vi "Ivium driver 1-03 - Copy2.vi"() -> ()   [LabVIEW 2020]
uses:
  Users/Benjamin/Desktop/StateMachine/Documents/LabVIEW Data/transmittance/controls/State.ctl
  IVIUM_remdriver.lvlib
panel:
  in  "Get device status 2":bool
  in  "Tab Control Ac/external/bistat":enum32{"AC", "Extern", "BiStat"}(tab)
  in  "Record I":bool
  in  "Read and set values":bool
  in  "Exit and disconnect":bool
  out "Values to re-intialise to at end\nof the measument":T1
  out "Device serial number":string
  in  "Read device serial number":bool
  in  "Tab Control direct mode/method mode":enum32{"Direct Control", "Method control"}(tab)
  out "cell on":bool
  in  "Set Mux channel":i32
  in  "Get current":bool
  out "current":dbl caption="A" format="%_4g"
  in  "cell potential":dbl caption="V" format="%_3p"
  in  "Apply":enum16{"off", "on"}(ring)
  in  "Current range":T2(ring)=enum."10 mA"
  in  "Configuration":T3(ring)
  out "Device Status indicator":string
  in  "Get device status":bool
  out "cell-off button pressed":bool
  out "E_overload":bool
  out "Aninput1_overload":bool
  out "I_overload":bool
  in  "Get cell status":bool
  in  "Reset 2":bool
  out "potential":dbl caption="V" format="%_4g"
  in  "Get potential":bool
  in  "Set Filter":T4(ring)=enum."10 kHz"
  in  "Set Stability":T5(ring)=enum."Standard"
  in  "Reset 3":bool
  in  "stop":bool
  # "Ac signal"
  # "Analog input"
  # "Digital output"
  # "Analog output"
  # "ch1"
  # "ch2"
  # "ch3"
  # "ch4"
  # "ch5"
  # "Digital input"
  # "ch6"
  # "ch7"
  # "ch8"
  # "I overload"
  # "Cell-off button pressed"
  # "E overload"
  # "Aninput1 overload"
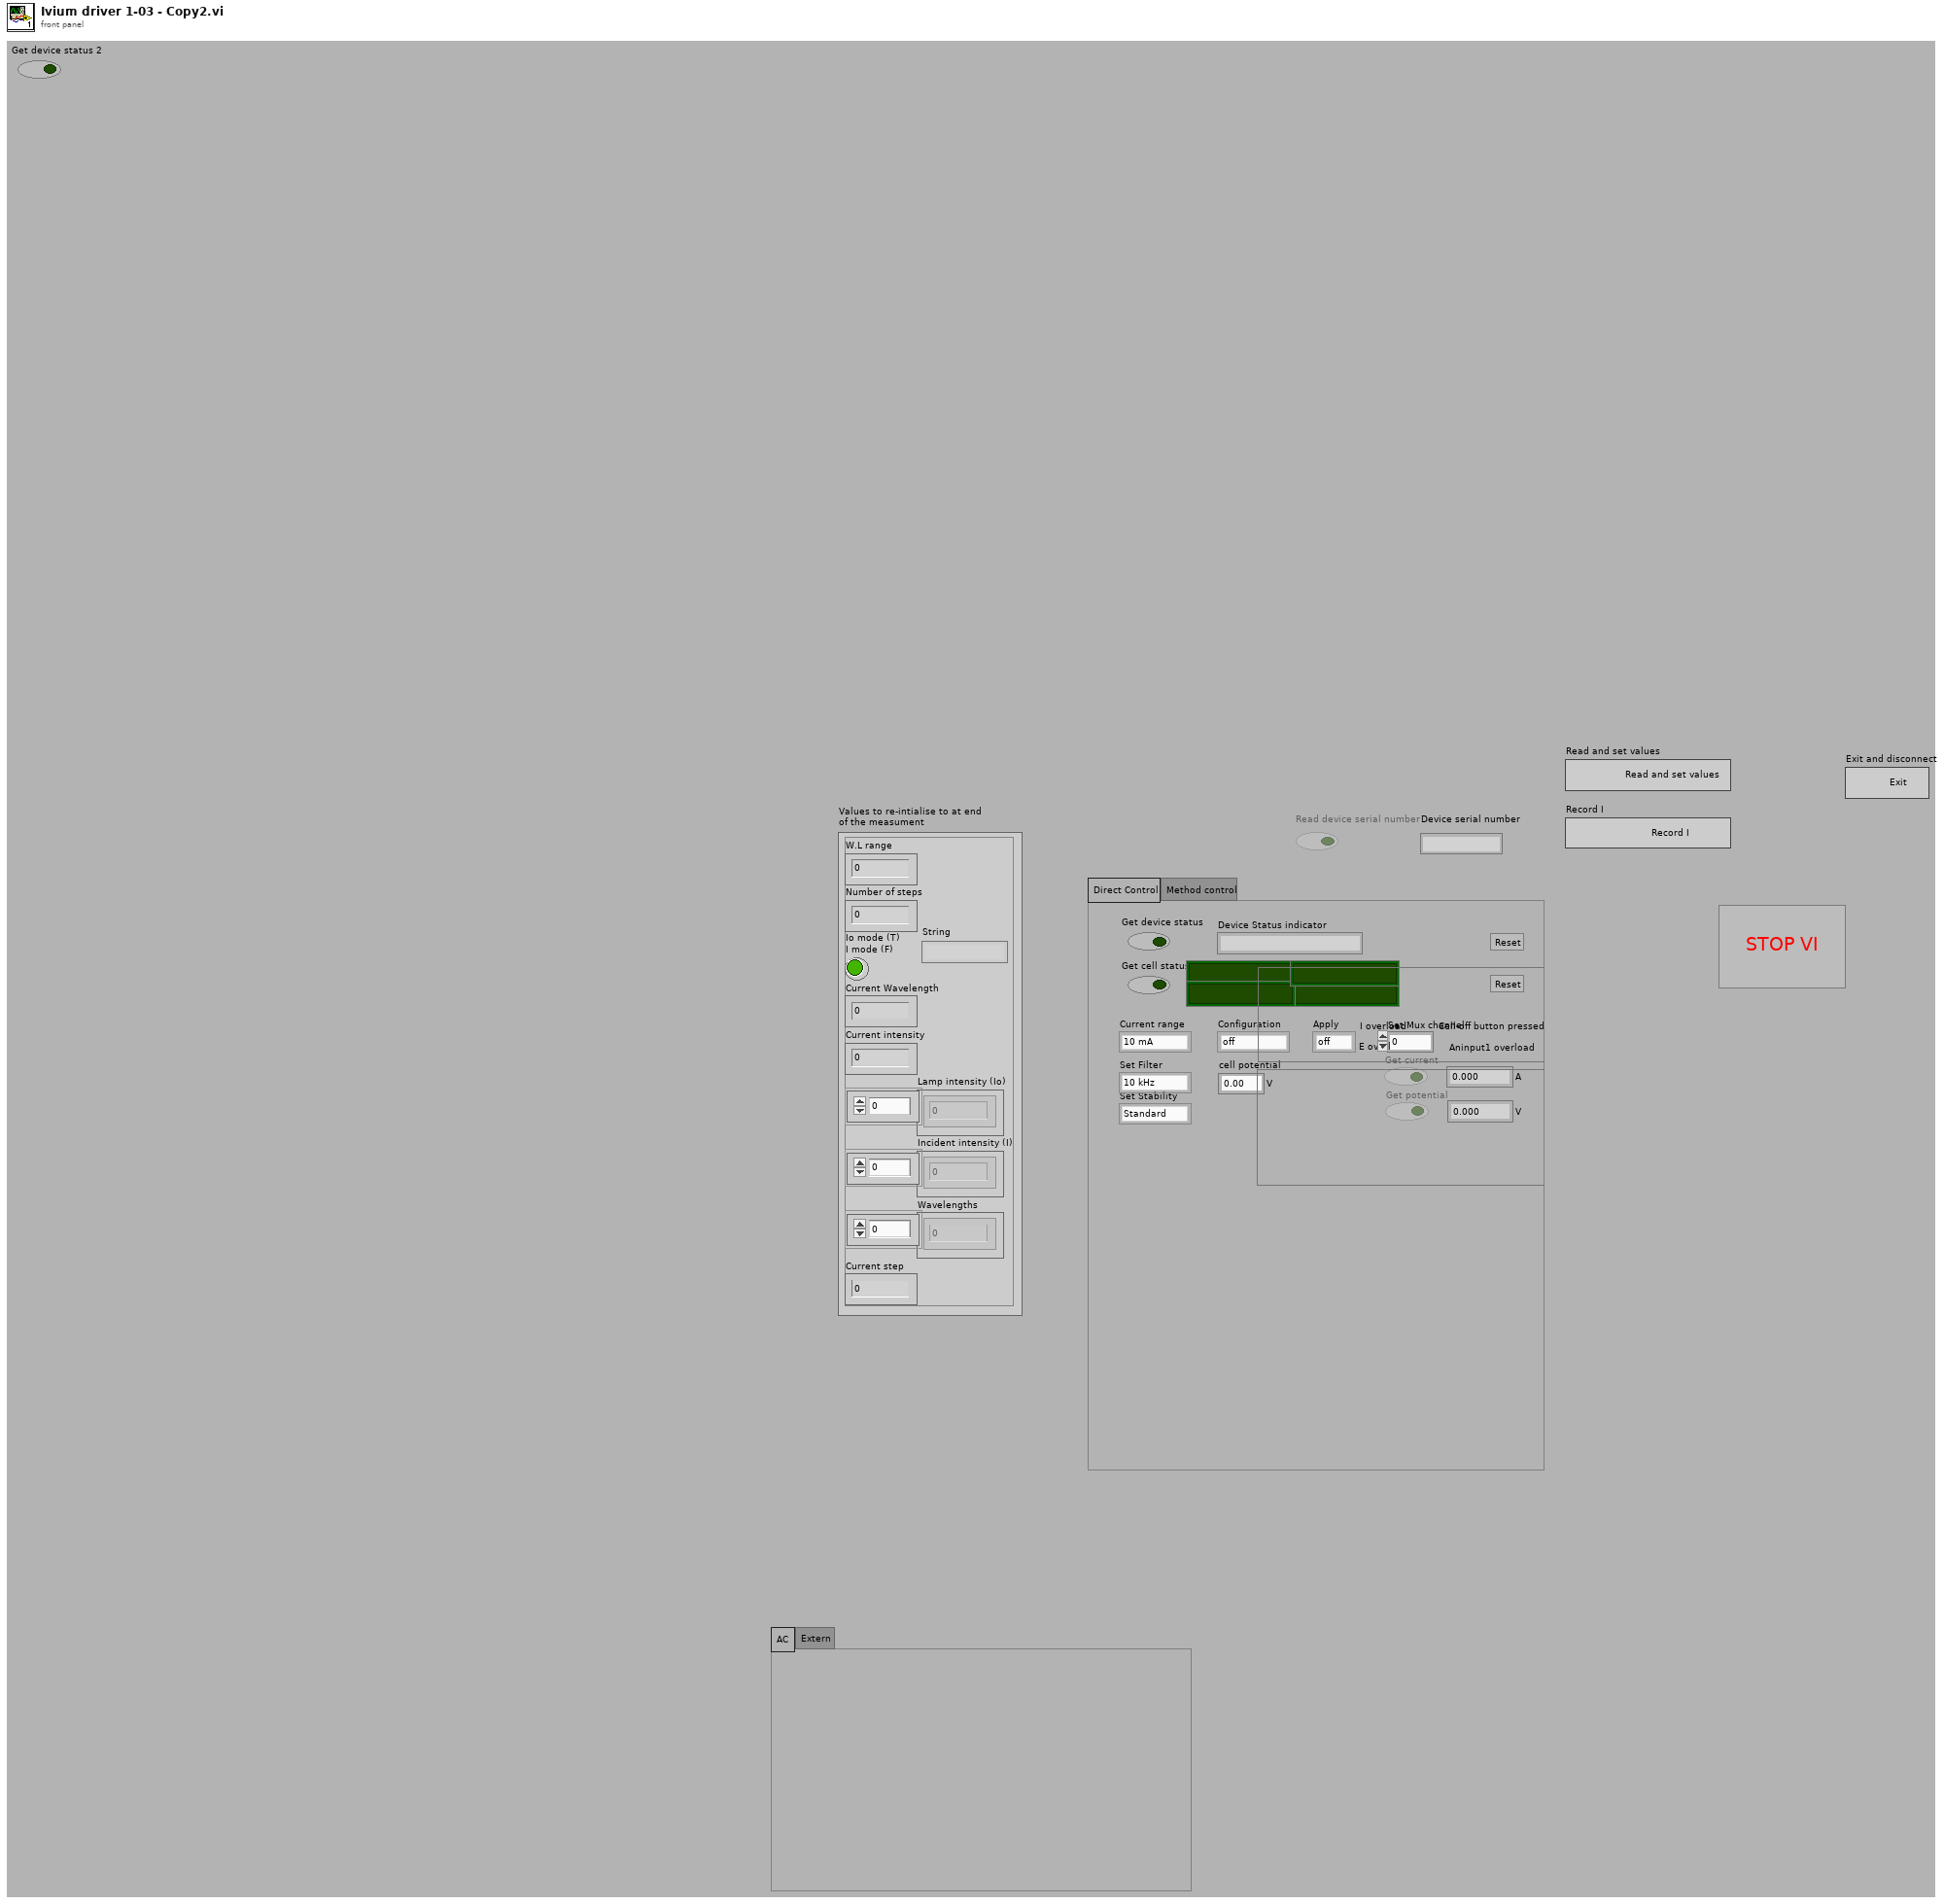
[diagram p1: front panel]
types:
  T1 = cluster{"W.L range":dbl, "Number of steps":dbl, "Io mode (T) \nI mode (F)":bool, "Current Wavelength":dbl, "Current intensity":dbl, "Lamp intensity (Io)":dbl[], "Incident intensity (I) ":dbl[], "Wavelengths ":dbl[], "Current step":dbl, "String":string}
  T2 = enum16{"10 A", "1 A", "100 mA", "10 mA", "1 mA", "100 uA", "10 uA", "1 uA", "100 nA", "10 nA", "1 nA", "100 pA", "10 pA", "1 pA"}
  T3 = enum16{"off", "EStat4EL", "EStat2EL", "EStatDummy1", "EStatDummy2", "EStatDummy3", "EStatDummy4", "IStat4EL", "IStat2EL", "IStatDummy", "BiStat4EL", "BiStat2EL"}
  T4 = enum16{"1 MHz", "100 kHz", "10 kHz", "1 kHz", "10 Hz"}
  T5 = enum16{"High Speed", "Standard", "High Stability"}
  T6 = cluster{"W.L range":dbl, "Number of steps":dbl, "Io mode (T) \nI mode (F)":bool, "Current Wavelength":dbl, "Current intensity":dbl, "Lamp intensity (Io)":dbl[], "Incident intensity (I) ":dbl[], "Wavelengths ":dbl[], "Current step":dbl, "Status":string}
  T7 = typedef "State.ctl" = enum16{"Initialize", "Wait for Event", "Update and read", "Close ", "Output data and process", "Exit"}
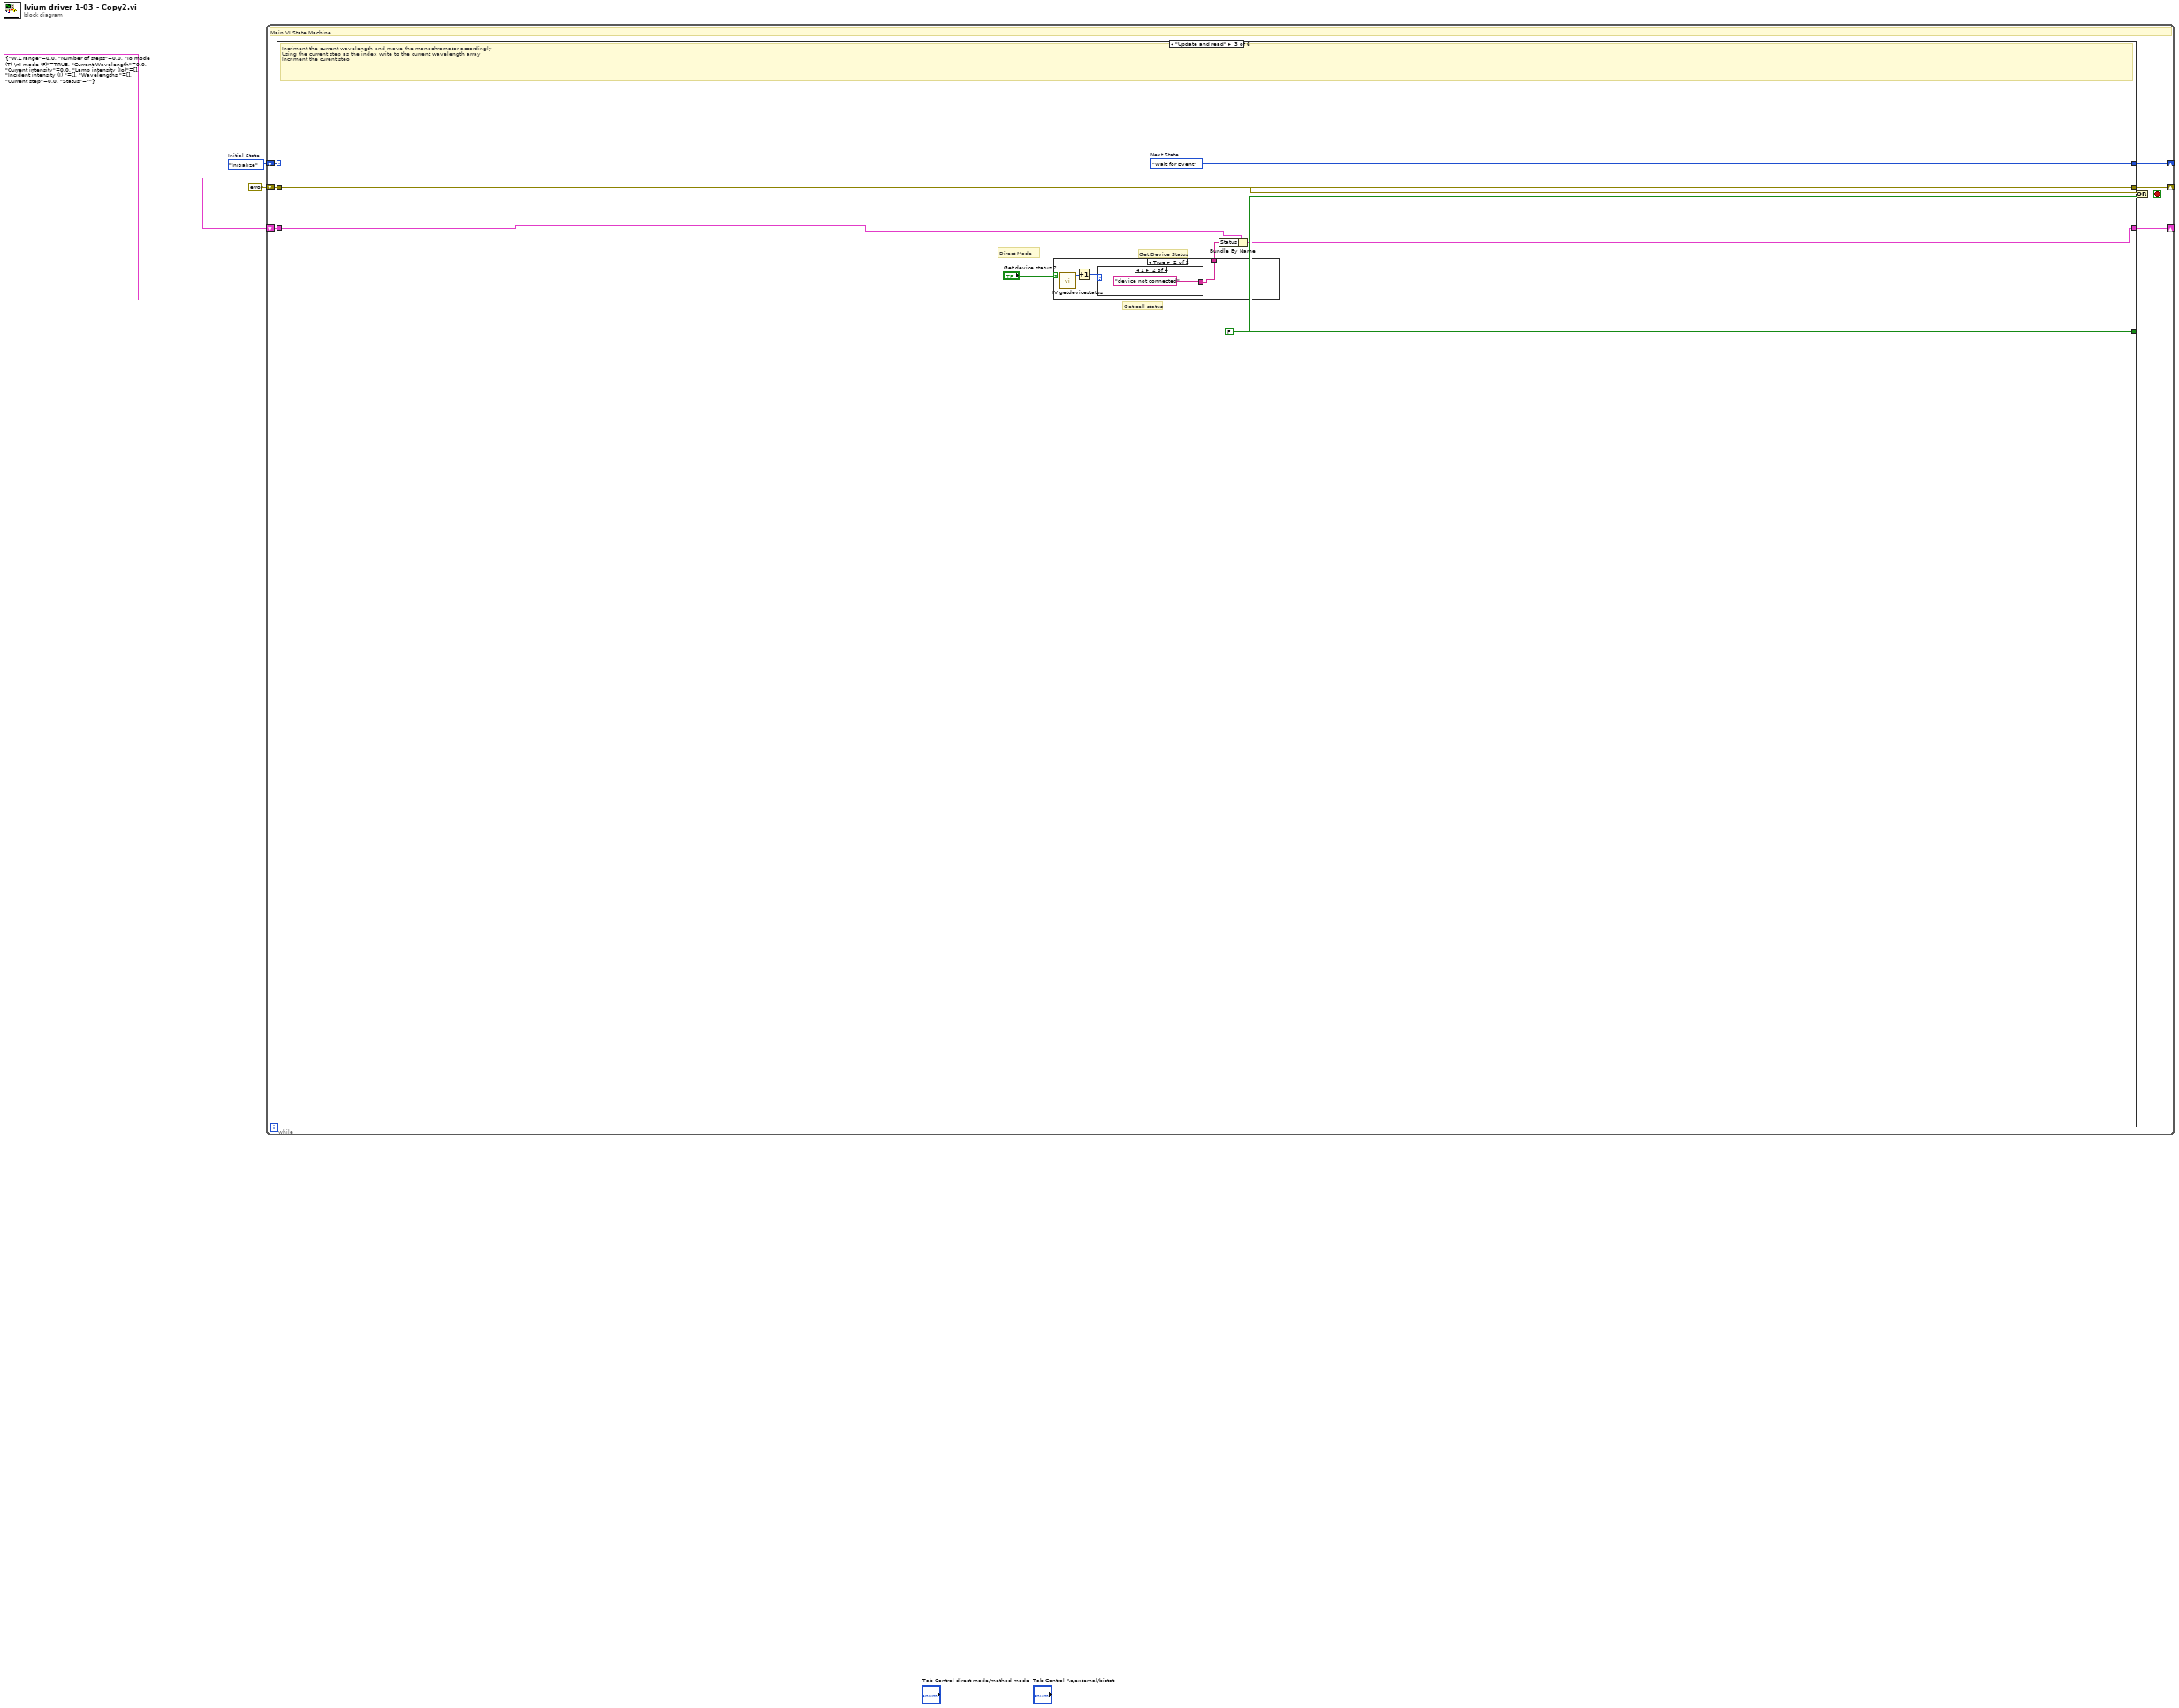
[diagram p0: block diagram]
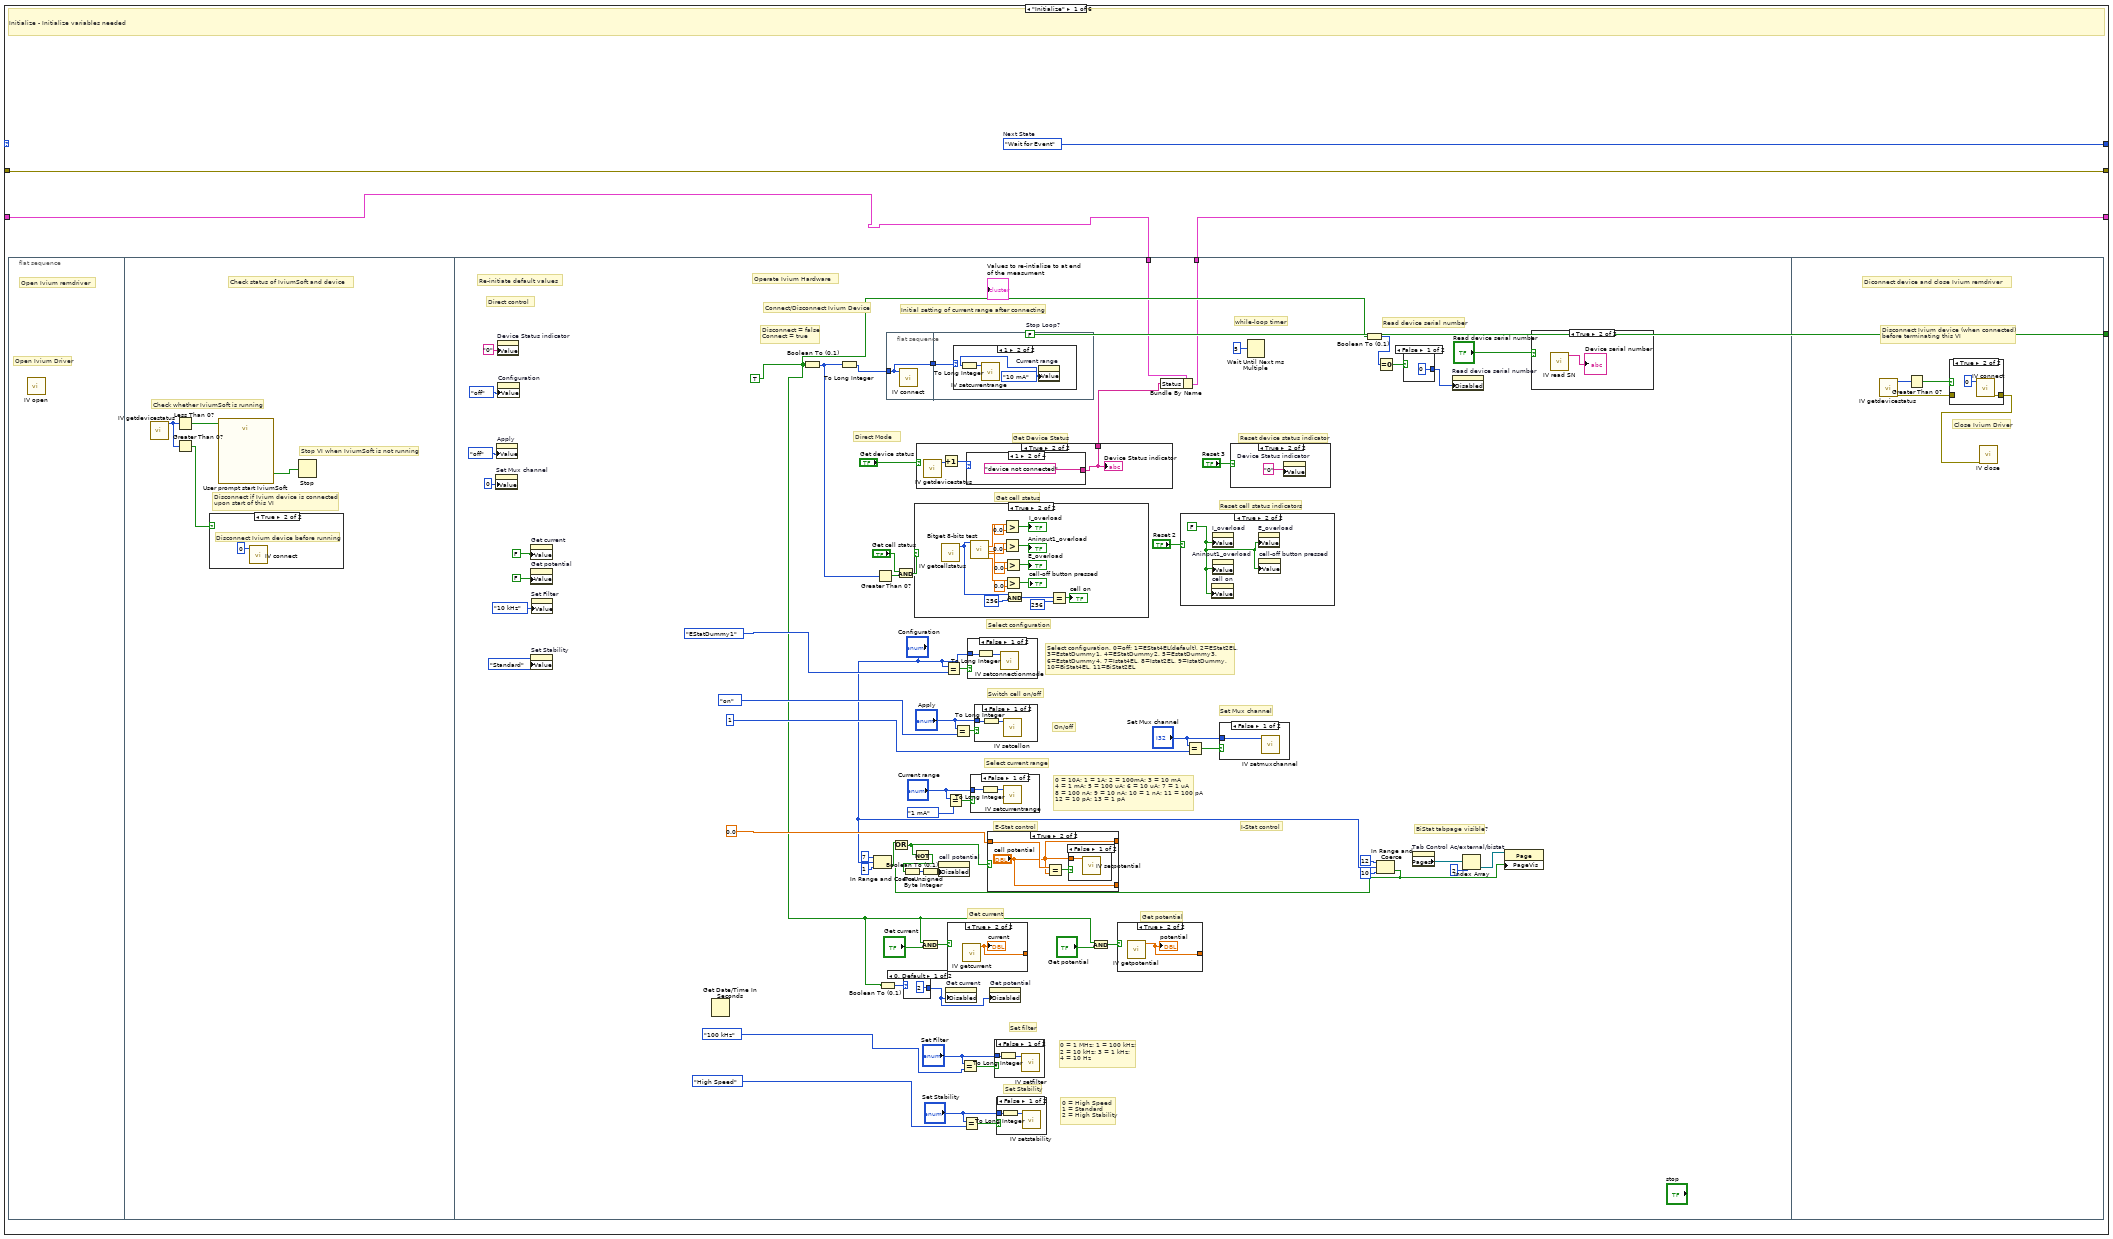
[diagram p2: hidden frame]
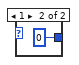
[diagram p5: hidden frame]
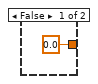
[diagram p10: hidden frame]
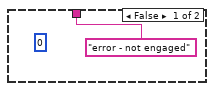
[diagram p13: hidden frame]
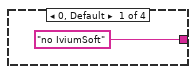
[diagram p14: hidden frame]
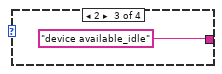
[diagram p15: hidden frame]
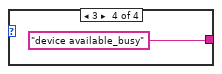
[diagram p16: hidden frame]
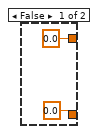
[diagram p17: hidden frame]
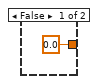
[diagram p19: hidden frame]
diagram:
  w3 = State."Initialize"  # Initial State
  n1 = while {
    shift-right: [w10] -> _
    shift-left: w3 -> [w11]
    shift-right: [w8] -> _
    shift-left: T6 {"W.L range"=0.0, "Number of steps"=0.0, "Io mode (T) \nI mode (F)"=TRUE, "Current Wavelength"=0.0, "Current intensity"=0.0, "Lamp intensity (Io)"=[], "Incident intensity (I) "=[], "Wavelengths "=[], "Current step"=0.0, "Status"=""} -> [w9]
    shift-right: [w4] -> _
    shift-left: errorcluster {"status"=FALSE, "code"=0, "source"=""} ("error constant") -> [w7]
    stop <- w5 stop-if-true
    # "Main VI State Machine"
    n2 = case shown="\"Update and read\"" w11 {
      tunnel: [w16 w155 w175 w192 State."Exit" ("f") State."Wait for Event" ("f")] -> w10
      tunnel: [w15 w154 FALSE ("Stop Loop?") w190 _ _] -> w6
      tunnel: w9 -> [w12 w151 w171 w191 w198 _]
      tunnel: [w13 w150 w169 w191 w198 w199] -> w8
      tunnel: w7 -> [w14 w153 w173 w185 w197 w201]
      tunnel: [w14 w152 w173 w184 w197 w201] -> w4
      frame "Initialize" {
        w15 = FALSE  # Stop Loop?
        w16 = State."Wait for Event"  # Next State
        # "Initialize - Initialize variables needed"
        n3 = flat-sequence {
          tunnel: w12 -> [w24]
          tunnel: [w22] -> w13
          frame #0 {
            # "Open Ivium Driver"
            # "Open Ivium remdriver"
            n4 = call "IV open.vi"() -> ()  [unwired: 10 in, 2 out]
          }
          frame #1 {
            # "Check status of IviumSoft and device"
            # "Stop VI when IviumSoft is not running"
            # "Disconnect if Ivium device is connected \nupon start of this VI"
            # "Check whether IviumSoft is running"
            n5 = call "IV getdevicestatus.vi"() -> ("return type"=w20:i32)  [unwired: 10 in, 1 out]
            n6 = Less Than 0?(x=w20) -> (x < 0?=w17:bool)
            n7 = Greater Than 0?(x=w20) -> (x > 0?=w19:bool)
            n8 = case shown="True" w19 {
              frame False {
              }
              frame True {
                # "Disconnect Ivium device before running"
                n9 = call "IV connect.vi"("devconnect"=0) -> ()  [unwired: 8 in, 3 out]
              }
            }
            n10 = call "User prompt start IviumSoft.vi"("Enable"=w17) -> ("OK"=w18:bool)  [unwired: 17 in, 1 out]
            n11 = Stop(stop? (T)=w18) -> ()
          }
          frame #2 {
            w26 = TRUE ("Boolean")
            # "BiStat tabpage visible?"
            # "Get potential"
            # "Get current"
            # "Set Mux channel"
            # "Reset device status indicator"
            # "0 = High Speed\n1 = Standard \n2 = High Stability"
            # "Set Stability"
            # "0 = 1 MHz; 1 = 100 kHz; \n2 = 10 kHz; 3 = 1 kHz; \n4 = 10 Hz"
            # "Set filter"
            # "On/off"
            # "I-Stat control"
            # "E-Stat control"
            # "Reset cell status indicators"
            # "Get cell status"
            # "Get Device Status"
            # "0 = 10A; 1 = 1A; 2 = 100mA; 3 = 10 mA\n4 = 1 mA; 5 = 100 uA; 6 = 10 uA; 7 = 1 uA\n8 = 100 nA; 9 = 10 nA; 10 = 1 nA; 11 = 100 pA\n12 = 10 pA; 13 = 1 pA"
            # "Select configuration"
            # "Direct Mode"
            # "Switch cell on/off"
            # "Select current range"
            # "Select configuration, 0=off; 1=EStat4EL(default), 2=EStat2EL, 3=EstatDummy1, 4=EStatDummy2, 5=EstatDummy3, 6=EstatDummy4, 7=Istat4EL, 8=Istat2EL, 9=IstatDummy, 10=BiStat4EL, 11=BiStat2EL"
            # "Read device serial number"
            # "while-loop timer"
            # "Initial setting of current range after connecting"
            # "Disconnect = false\nConnect = true"
            # "Connect/Disconnect Ivium Device"
            # "Direct control"
            # "Re-initiate default values"
            # "Operate Ivium Hardware"
            n12 = property on="Set Mux channel" class="DigNum (strict)"("Value"=0 ("Set Mux channel")) -> ()  [unwired: 2 in, 2 out]
            n13 = property on="Apply" class="Enum (strict)"("Value"=enum16{"off", "on"}."off" ("Cell on/off")) -> ()  [unwired: 2 in, 2 out]
            n14 = property on="Device Status indicator" class="Str"("Value"="0" ("Device Status indicator 2")) -> ()  [unwired: 2 in, 2 out]
            n15 = property on="Configuration" class="Enum (strict)"("Value"=T3."off" ("Configuration")) -> ()  [unwired: 2 in, 2 out]
            n16 = property on="Get current" class="Bool (strict)"("Value"=FALSE ("Get current")) -> ()  [unwired: 2 in, 2 out]
            n17 = property on="Get potential" class="Bool (strict)"("Value"=FALSE ("Get potential")) -> ()  [unwired: 2 in, 2 out]
            n18 = property on="Set Stability" class="Enum (strict)"("Value"=T5."Standard" ("Set Stability")) -> ()  [unwired: 2 in, 2 out]
            n19 = property on="Set Filter" class="Enum (strict)"("Value"=T4."10 kHz" ("Set Filter")) -> ()  [unwired: 2 in, 2 out]
            n20 = Get Date/Time In Seconds() -> ()  [unwired: 1 out]
            n21 = Boolean To (0,1)(Boolean=w26) -> (0, 1=w69:i16)
            n22 = To Long Integer(number=w69) -> (32bit integer=w70:i32)
            n23 = In Range and Coerce(upper limit=u16 7, x="Configuration", lower limit=u16 1) -> (In Range?=w47:bool)  [unwired: 1 out]
            n24 = Greater Than 0?(x=w69) -> (x > 0?=w51:bool)
            n25 = Boolean To (0,1)(Boolean=w26) -> (0, 1=w39:i16)
            n26 = flat-sequence {
              tunnel: w70 -> [w86]
              tunnel: [w86] -> w25
              tunnel: w25 -> [w87]
              frame #0 {
                n27 = call "IV connect.vi"("devconnect"=w86) -> ()  [unwired: 8 in, 3 out]
              }
              frame #1 {
                n28 = case shown="1" w87 {
                  frame 0, Default {
                  }
                  frame 1 {
                    w88 = T2."10 mA" ("Current range selector")
                    n29 = To Long Integer(number=w88) -> (32bit integer=w89:i32)
                    n30 = call "IV setcurrentrange.vi"("value"=w89) -> ()  [unwired: 8 in, 3 out]
                    n31 = property on="Current range" class="Enum (strict)"("Value"=w88) -> ()  [unwired: 2 in, 2 out]
                  }
                }
              }
            }
            n32 = And(x="Get cell status", y=w51) -> (x .and. y?=w53:bool)
            n33 = case shown="0, Default" w39 {
              tunnel: [u8 2 u8 0] -> w38
              frame 0, Default {
              }
              frame 1 {
              }
            }
            n34 = case shown="True" w53 {
              frame False {
              }
              frame True {
                n35 = call "IV getcellstatus.vi"() -> ("devcellstatus out"=w105:i32)  [unwired: 9 in, 2 out]
                n36 = call "Bitget 8-bits test.vi"("x"=w105) -> ("c"=w110:dbl, "e"=w108:dbl, "f"=w109:dbl, "h"=w106:dbl)  [unwired: 19 in, 4 out]
                n37 = Greater?(x=w110, y=0.0) -> (0:→"I_overload":bool)
                n38 = Greater?(x=w108, y=0.0) -> (0:→"Aninput1_overload":bool)
                n39 = Greater?(x=w109, y=0.0) -> (0:→"E_overload":bool)
                n40 = Greater?(x=w106, y=0.0) -> (0:→"cell-off button pressed":bool)
                n41 = And(x=w105, y=256) -> (x .and. y?=w103:i32)
                n42 = Equal?(x=w103, y=256) -> (x = y?=→"cell on":bool)
              }
            }
            n43 = case shown="True" "Get device status" {
              tunnel: ["error - not engaged" w119] -> w23
              frame False {
                (unwired) 0
              }
              frame True {
                n44 = call "IV getdevicestatus.vi"() -> ("return type"=w121:i32)  [unwired: 10 in, 1 out]
                n45 = Increment(x=w121) -> (x+1=w120:i32)
                n46 = case shown="1" w120 {
                  tunnel: ["no IviumSoft" "device not connected" "device available_idle" "device available_busy"] -> w119
                  frame 0, Default {
                  }
                  frame 1 {
                  }
                  frame 2 {
                  }
                  frame 3 {
                  }
                }
                "Device Status indicator" <- w119
              }
            }
            n47 = And(x=w26, y="Get current") -> (x .and. y?=w60:bool)
            n48 = Equal?(x="Configuration", y=T3."EStatDummy1" ("Configuration")) -> (x = y?=w63:bool)
            n49 = property on="Get current" class="Bool (strict)"("Disabled"=w38) -> ()  [unwired: 2 in, 2 out]
            n50 = Equal?(x="Current range", y=T2."1 mA") -> (x = y?=w64:bool)
            n51 = case shown="True" w60 {
              tunnel: [0.0 ("value out") w133] -> _
              frame False {
              }
              frame True {
                n52 = call "IV getcurrent.vi"() -> ("value out"=w133:dbl)  [unwired: 9 in, 2 out]
                "current" <- w133
              }
            }
            n53 = Equal?(x="Apply", y=enum16{"off", "on"}."on" ("Apply")) -> (x = y?=w62:bool)
            n54 = Equal?(x="Set Filter", y=T4."100 kHz" ("Set Filter")) -> (x = y?=w31:bool)
            n55 = Equal?(x="Set Stability", y=T5."High Speed" ("Set Stability")) -> (x = y?=w44:bool)
            n56 = case shown="False" w63 {
              tunnel: "Configuration" -> [w136 _]
              frame False {
                n57 = To Long Integer(number=w136) -> (32bit integer=w137:i32)
                n58 = call "IV setconnectionmode.vi"("value"=w137) -> ()  [unwired: 8 in, 3 out]
              }
              frame True {
              }
            }
            n59 = case shown="False" w64 {
              tunnel: "Current range" -> [w138 _]
              frame False {
                n60 = To Long Integer(number=w138) -> (32bit integer=w139:i32)
                n61 = call "IV setcurrentrange.vi"("value"=w139) -> ()  [unwired: 8 in, 3 out]
              }
              frame True {
              }
            }
            n62 = case shown="False" w62 {
              tunnel: "Apply" -> [w134 _]
              frame False {
                n63 = To Long Integer(number=w134) -> (32bit integer=w135:i32)
                n64 = call "IV setcellon.vi"("cellon"=w135) -> ()  [unwired: 8 in, 3 out]
              }
              frame True {
              }
            }
            n65 = property on="Get potential" class="Bool (strict)"("Disabled"=w38) -> ()  [unwired: 2 in, 2 out]
            n66 = case shown="False" w31 {
              tunnel: "Set Filter" -> [w97 _]
              frame False {
                n67 = To Long Integer(number=w97) -> (32bit integer=w96:i32)
                n68 = call "IV setfilter.vi"("value"=w96) -> ()  [unwired: 8 in, 3 out]
              }
              frame True {
              }
            }
            n69 = case shown="False" w44 {
              tunnel: "Set Stability" -> [w95 _]
              frame False {
                n70 = To Long Integer(number=w95) -> (32bit integer=w94:i32)
                n71 = call "IV setstability.vi"("value"=w94) -> ()  [unwired: 8 in, 3 out]
              }
              frame True {
              }
            }
            n72 = And(x=w26, y="Get potential") -> (x .and. y?=w46:bool)
            n73 = case shown="True" w46 {
              tunnel: [0.0 ("value out") w99] -> _
              frame False {
              }
              frame True {
                n74 = call "IV getpotential.vi"() -> ("value out"=w99:dbl)  [unwired: 9 in, 2 out]
                "potential" <- w99
              }
            }
            n75 = Bundle By Name(cluster=w24, "Status"=w23) -> (w22:T6)
            n76 = case shown="True" "Reset 2" {
              frame False {
              }
              frame True {
                w100 = FALSE
                n77 = property on="cell on" class="Bool (strict)"("Value"=w100) -> ()  [unwired: 2 in, 2 out]
                n78 = property on="I_overload" class="Bool (strict)"("Value"=w100) -> ()  [unwired: 2 in, 2 out]
                n79 = property on="Aninput1_overload" class="Bool (strict)"("Value"=w100) -> ()  [unwired: 2 in, 2 out]
                n80 = property on="E_overload" class="Bool (strict)"("Value"=w100) -> ()  [unwired: 2 in, 2 out]
                n81 = property on="cell-off button pressed" class="Bool (strict)"("Value"=w100) -> ()  [unwired: 2 in, 2 out]
              }
            }
            n82 = Equal?(x="Set Mux channel", y=1 ("Set Mux channel")) -> (x = y?=w42:bool)
            n83 = case shown="False" w42 {
              tunnel: "Set Mux channel" -> [w92 _]
              frame False {
                n84 = call "IV setmuxchannel.vi"("value"=w92) -> ()  [unwired: 8 in, 3 out]
              }
              frame True {
              }
            }
            n85 = case shown="True" "Reset 3" {
              frame False {
              }
              frame True {
                n86 = property on="Device Status indicator" class="Str"("Value"="0" ("Device Status indicator")) -> ()  [unwired: 2 in, 2 out]
              }
            }
            n87 = Wait Until Next ms Multiple(millisecond multiple=u32 5 ("milliseconds to wait")) -> ()  [unwired: 1 out]
            n88 = Boolean To (0,1)(Boolean=w26) -> (0, 1=w68:i16)
            n89 = In Range and Coerce(upper limit=u16 12, x="Configuration", lower limit=u16 10) -> (In Range?=w30:bool)  [unwired: 1 out]
            n90 = Or(x=w47, y=w30) -> (x .or. y?=w29:bool)
            n91 = Not(x=w29) -> (.not. x?=w55:bool)
            n92 = Boolean To (0,1)(Boolean=w55) -> (0, 1=w36:i16)
            n93 = To Unsigned Byte Integer(number=w36) -> (unsigned 8bit integer=w37:u8)
            n94 = property on="cell potential" class="DigNum (strict)"("Disabled"=w37) -> ()  [unwired: 2 in, 2 out]
            n95 = case shown="True" w29 {
              tunnel: [0.0 ("cell potential") "cell potential"] -> _
              tunnel: 0.0 -> [_ w129]
              tunnel: [0.0 ("cell potential") "cell potential"] -> _
              frame False {
              }
              frame True {
                n96 = Equal?(x=w129, y="cell potential") -> (x = y?=w130:bool)
                n97 = case shown="False" w130 {
                  tunnel: "cell potential" -> [w131 _]
                  frame False {
                    n98 = call "IV setpotential.vi"("value"=w131) -> ()  [unwired: 8 in, 3 out]
                  }
                  frame True {
                  }
                }
              }
            }
            n99 = Equal To 0?(x=w68) -> (x = 0?=w67:bool)
            n100 = case shown="False" w67 {
              tunnel: [u8 0 u8 2] -> w66
              frame False {
              }
              frame True {
              }
            }
            n101 = property on="Tab Control Ac/external/bistat" class="TabCtl (strict)"() -> ("Pages"=w34:refnum<vi>[])  [unwired: 2 in, 2 out]
            n102 = property on="Read device serial number" class="Bool"("Disabled"=w66) -> ()  [unwired: 2 in, 2 out]
            n103 = Index Array(array=w34, index=2) -> (element=w32:refnum<vi>)
            n104 = property class="Page"(reference=w32, "PageVis"=w30) -> ()  [unwired: 1 in, 2 out]
            n105 = case shown="True" "Read device serial number" {
              frame False {
              }
              frame True {
                n106 = call "IV read SN.vi"() -> ("sntext out"=→"Device serial number":string)  [unwired: 9 in, 2 out]
              }
            }
          }
          frame #3 {
            # "Diconnect device and close Ivium remdriver"
            # "Disconnect Ivium device (when connected)\nbefore terminating this VI"
            # "Close Ivium Driver"
            n107 = call "IV getdevicestatus.vi"() -> ("error out"=w143:errorcluster, "return type"=w145:i32)  [unwired: 10 in]
            n108 = Greater Than 0?(x=w145) -> (x > 0?=w144:bool)
            n109 = case shown="True" w144 {
              tunnel: [w147 w148] -> w146
              tunnel: w143 -> [w147 _]
              frame False {
              }
              frame True {
                n110 = call "IV connect.vi"("devconnect"=0) -> ("error out"=w148:errorcluster)  [unwired: 8 in, 2 out]
              }
            }
            n111 = call "IV close.vi"("error in (no error)"=w146) -> ()  [unwired: 9 in, 2 out]
          }
        }
      }
      frame "Wait for Event" {
        w154 = FALSE  # Stop Loop?
        # "Wait for Event - Use an Event Structure to monitor the user interface for events that run different states of the state machine."
        n112 = event shown="[1] \"Read and set values\": Value Change" {
          selector: _ -> [_ _ _]
          dyn-events: _ -> [_ _ _]
          timeout: _ -> [_ _ _]
          tunnel: [w158 w162 w168] -> w155
          tunnel: [w156 w159 w164] -> w150
          tunnel: w153 -> [w157 w163 w167]
          tunnel: [w157 w163 w167] -> w152
          tunnel: w151 -> [w156 w161 w165]
          event "Exit and disconnect": Value Change {
            w158 = State."Exit"  # Next State
            n113 = event-data() -> ()  [unwired: 1 in, 1 out]
          }
          event "Read and set values": Value Change {
            w162 = State."Update and read"  # Initial State
            n114 = event-data() -> ()  [unwired: 1 in, 1 out]
            n115 = Bundle By Name(cluster=w161, "Io mode (T) \nI mode (F)"=TRUE) -> (w159:T6)
          }
          event "Record I": Value Change {
            w168 = State."Close "  # Next State
            # "Here, I or Io modes is chosen."
            n116 = event-data() -> ()  [unwired: 1 in, 1 out]
            n117 = Bundle By Name(cluster=w165, "Io mode (T) \nI mode (F)"=FALSE) -> (w164:T6)
          }
        }
      }
      frame "Update and read" {
        w175 = State."Wait for Event"  # Next State
        # "Get cell status"
        # "Get Device Status"
        # "Direct Mode"
        # "Incriment the current wavelength and move the monochromator accordingly\nUsing the current step as the index write to the current wavelength array\nIncriment the curent steo"
        n118 = case shown="True" "Get device status 2" {
          tunnel: ["error - not engaged" w177] -> w170
          frame False {
            (unwired) 0
          }
          frame True {
            n119 = call "IV getdevicestatus.vi"() -> ("return type"=w179:i32)  [unwired: 10 in, 1 out]
            n120 = Increment(x=w179) -> (x+1=w178:i32)
            n121 = case shown="1" w178 {
              tunnel: ["no IviumSoft" "device not connected" "device available_idle" "device available_busy"] -> w177
              frame 0, Default {
              }
              frame 1 {
              }
              frame 2 {
              }
              frame 3 {
              }
            }
          }
        }
        n122 = Bundle By Name(cluster=w171, "Status"=w170) -> (w169:T6)
      }
      frame "Exit" {
        w190 = TRUE  # Stop Loop?
        w192 = State."Exit"  # (Value Not Used)
        # "Diconnect device and close Ivium remdriver"
        # "Disconnect Ivium device (when connected)\nbefore terminating this VI"
        # "Close Ivium Driver"
        # "Exit - Exit the application."
        n123 = call "IV getdevicestatus.vi"("error in (no error)"=w185) -> ("error out"=w186:errorcluster, "return type"=w188:i32)  [unwired: 9 in]
        n124 = Greater Than 0?(x=w188) -> (x > 0?=w187:bool)
        n125 = case shown="True" w187 {
          tunnel: [w193 w194] -> w189
          tunnel: w186 -> [w193 _]
          frame False {
          }
          frame True {
            n126 = call "IV connect.vi"("devconnect"=0) -> ("error out"=w194:errorcluster)  [unwired: 8 in, 2 out]
          }
        }
        n127 = call "IV close.vi"("error in (no error)"=w189) -> ("error out"=w184:errorcluster)  [unwired: 9 in, 1 out]
      }
      frame "Close " {
      }
      frame "Output data and process" {
        # "Also re-intialise constants"
        n128 = local read "Values to re-intialise to at end\nof the measument"() -> (w199:T1)
      }
    }
    n129 = Or(x=w4, y=w6) -> (x .or. y?=w5:bool)
  }
